vi "init_delay_generator.vi"(5 "VISA resource name":refnum<visa-resource-name>) -> (0 "error out":errorcluster, 2 "VISA resource name out":refnum<visa-resource-name>)   [LabVIEW 2011]
doc: "Initializes the delay generator to the defaults settings, leaves the delay data untouched."
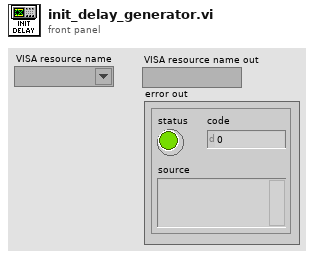
[diagram p1: front panel]
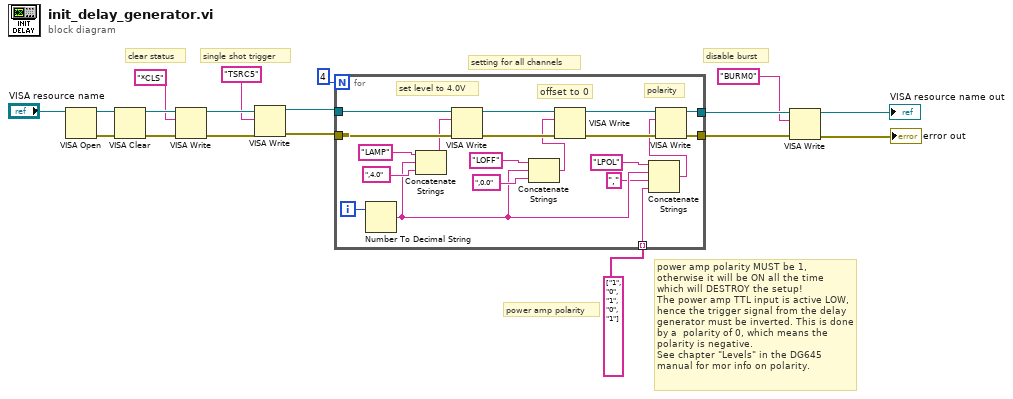
[diagram p0: block diagram]
diagram:
  # "power amp polarity"
  # "power amp polarity MUST be 1, \notherwise it will be ON all the time \nwhich will DESTROY the setup!\nThe power amp TTL input is active LOW,\nhence the trigger signal from the delay \ngenerator must be inverted. This is done \nby a  polarity of 0, which means the\npolarity is negative.\nSee chapter \"Levels\" in the DG645 \nmanual for mor info on polarity."
  # "setting for all channels"
  # "disable burst"
  # "clear status"
  # "single shot trigger"
  n1 = VISA Open(VISA resource name="VISA resource name") -> (VISA resource name=w17:refnum<visa-resource-name>, error out=w18:errorcluster)  [unwired: 4 in]
  n2 = VISA Clear(VISA resource name=w17, error in (no error)=w18) -> (VISA resource name out=w16:refnum<visa-resource-name>, error out=w15:errorcluster)
  n3 = VISA Write(VISA resource name=w16, write buffer="*CLS" ("Query 2"), error in (no error)=w15) -> (VISA resource name out=w12:refnum<visa-resource-name>, error out=w11:errorcluster)  [unwired: 1 out]
  n4 = VISA Write(VISA resource name=w12, write buffer="TSRC5" ("Query 2"), error in (no error)=w11) -> (VISA resource name out=w6:refnum<visa-resource-name>, error out=w4:errorcluster)  [unwired: 1 out]
  n5 = for {
    N: 4 -> [_]
    tunnel: w6 -> [w37]
    tunnel: [w24] -> w5
    tunnel: w4 -> [w36]
    tunnel: [w26] -> w3
    tunnel: string[] ["1", "0", "1", "0", "1"] ("polarity") -> [w20] mode=indexing
    i -> [w34]
    # "polarity"
    # "offset to 0"
    # "set level to 4.0V"
    n6 = Number To Decimal String(number=w34) -> (decimal integer string=w22:string)  [unwired: 1 in]
    n7 = Concatenate Strings("LAMP" ("Query 2"), w22, ",4.0" ("Query 2")) -> (w32:string)
    n8 = VISA Write(VISA resource name=w37, write buffer=w32, error in (no error)=w36) -> (VISA resource name out=w28:refnum<visa-resource-name>, error out=w35:errorcluster)  [unwired: 1 out]
    n9 = Concatenate Strings("LOFF" ("Query 2"), w22, ",0.0" ("Query 2")) -> (w27:string)
    n10 = VISA Write(VISA resource name=w28, write buffer=w27, error in (no error)=w35) -> (VISA resource name out=w25:refnum<visa-resource-name>, error out=w29:errorcluster)  [unwired: 1 out]
    n11 = Concatenate Strings("LPOL" ("Query 2"), w22, "," ("string"), w20) -> (w21:string)
    n12 = VISA Write(VISA resource name=w25, write buffer=w21, error in (no error)=w29) -> (VISA resource name out=w24:refnum<visa-resource-name>, error out=w26:errorcluster)  [unwired: 1 out]
  }
  n13 = VISA Write(VISA resource name=w5, write buffer="BURM0", error in (no error)=w3) -> (VISA resource name out=→"VISA resource name out":refnum<visa-resource-name>, error out=→"error out":errorcluster)  [unwired: 1 out]
